vi "ROI Descriptor.vi"(11 "Global Rectangle":i32[](array[numeric])=[27, 55, 270, 147]) -> (3 "ROI Descriptor":T1 {"Contours"."Type" items=["No Selection", "Point", "Line", "Rectangle", "Oval", "Polygon", "Free", "Annulus", "Unused2", "Unused3", "Broken Line", "Free Hand Line", "Rotated Rectangle"]})   [LabVIEW 2017]
panel:
  in  "ID":enum32{"External", "Internal"}(ring)
  in  "Type":u32(ring)=3 items=["No Selection", "Point", "Line", "Rectangle", "Oval", "Polygon", "Free", "Annulus", "Unused2", "Unused3", "Broken Line", "Free Hand Line", "Rotated Rectangle"]
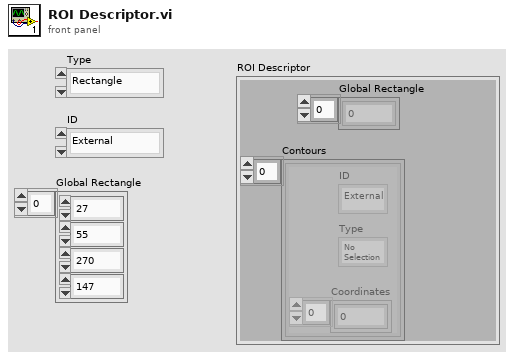
[diagram p1: front panel]
types:
  T1 = cluster{"Global Rectangle":i32[], "Contours":cluster{"ID":enum32{"External", "Internal"}, "Type":u32, "Coordinates":i32[]}[]}
  T2 = cluster{"ID":enum32{"External", "Internal"}, "Type":u32, "Global Rectangle":i32[]}
  T3 = cluster{"ID":enum32{"External", "Internal"}, "Type":u32, "Global Rectangle":i32[]}[]
  T4 = cluster{"Global Rectangle":i32[], cluster{"ID":enum32{"External", "Internal"}, "Type":u32, "Global Rectangle":i32[]}[]}
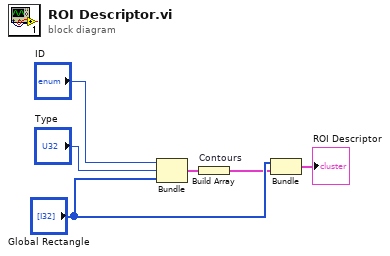
[diagram p0: block diagram]
diagram:
  n1 = Bundle("ID"="ID", "Type"="Type", "Global Rectangle"="Global Rectangle") -> (w6:T2)  [unwired: 1 in]
  n2 = Build Array "Contours"(w6) -> (w2:T3)
  n3 = Bundle("Global Rectangle"="Global Rectangle", w2) -> (→"ROI Descriptor":T4)  [unwired: 1 in]
